vi "Launcher.vi"() -> ()   [LabVIEW 2020]
uses:
  UI ACTOR.lvclass
  C:/Program Files (x86)/National Instruments/LabVIEW 2020/vi.lib/ActorFramework/Actor/Actor.lvclass
  HAL/Proyecto-Final/Implementations/Cypress/Cypress.lvclass
  C:/Users/danie/Desktop/LabView/3er Parcial/HAL/Proyecto-Final/Abstract/Serial Device/Serial Device.lvclass
  UI ACTOR.lvclass/UI ACTOR.ctl
  Write Serial Device.lvclass.vi
  <vilib>/ActorFramework/Actor/Actor.lvclass
panel:
  in  "Serial DEVICE":string(combo)
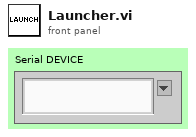
[diagram p1: front panel]
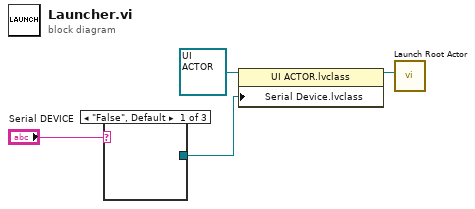
[diagram p0: block diagram]
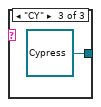
[diagram p3: hidden frame]
diagram:
  n1 = case shown="\"False\", Default" "Serial DEVICE" {
    tunnel: [_ _ refnum<class "Cypress.lvclass"> refnum ("Cypress.lvclass")] -> w2
    frame "False", Default {
    }
    frame "AR" {
    }
    frame "CY" {
    }
  }
  n2 = property class="UI ACTOR.lvclass"(reference=refnum<class "UI ACTOR.lvclass"> refnum ("UI ACTOR.lvlib:UI ACTOR.lvclass"), "Serial Device.lvclass"=w2) -> (reference out=w1:refnum<class "UI ACTOR.lvclass">)  [unwired: 1 in, 1 out]
  n3 = call <vilib>:"Launch Root Actor.vi"("Actor"=w1) -> ()  [unwired: 9 in, 2 out]
